vi "Stuck Key Parser.vi"(8 "error in (no error)":errorcluster, 10 "Numeric":u64, 11 "Parser Output Bundle":T1) -> (0 "error out":errorcluster, 3 "output cluster":T1)   [LabVIEW 2016]
panel:
  out "Group 7":bool[](array[boolean])
  out "Group 6":bool[](array[boolean])
  out "Group 5":bool[](array[boolean])
  out "Group 4":bool[](array[boolean])
  out "Group 3":bool[](array[boolean])
  out "Group 2":bool[](array[boolean])
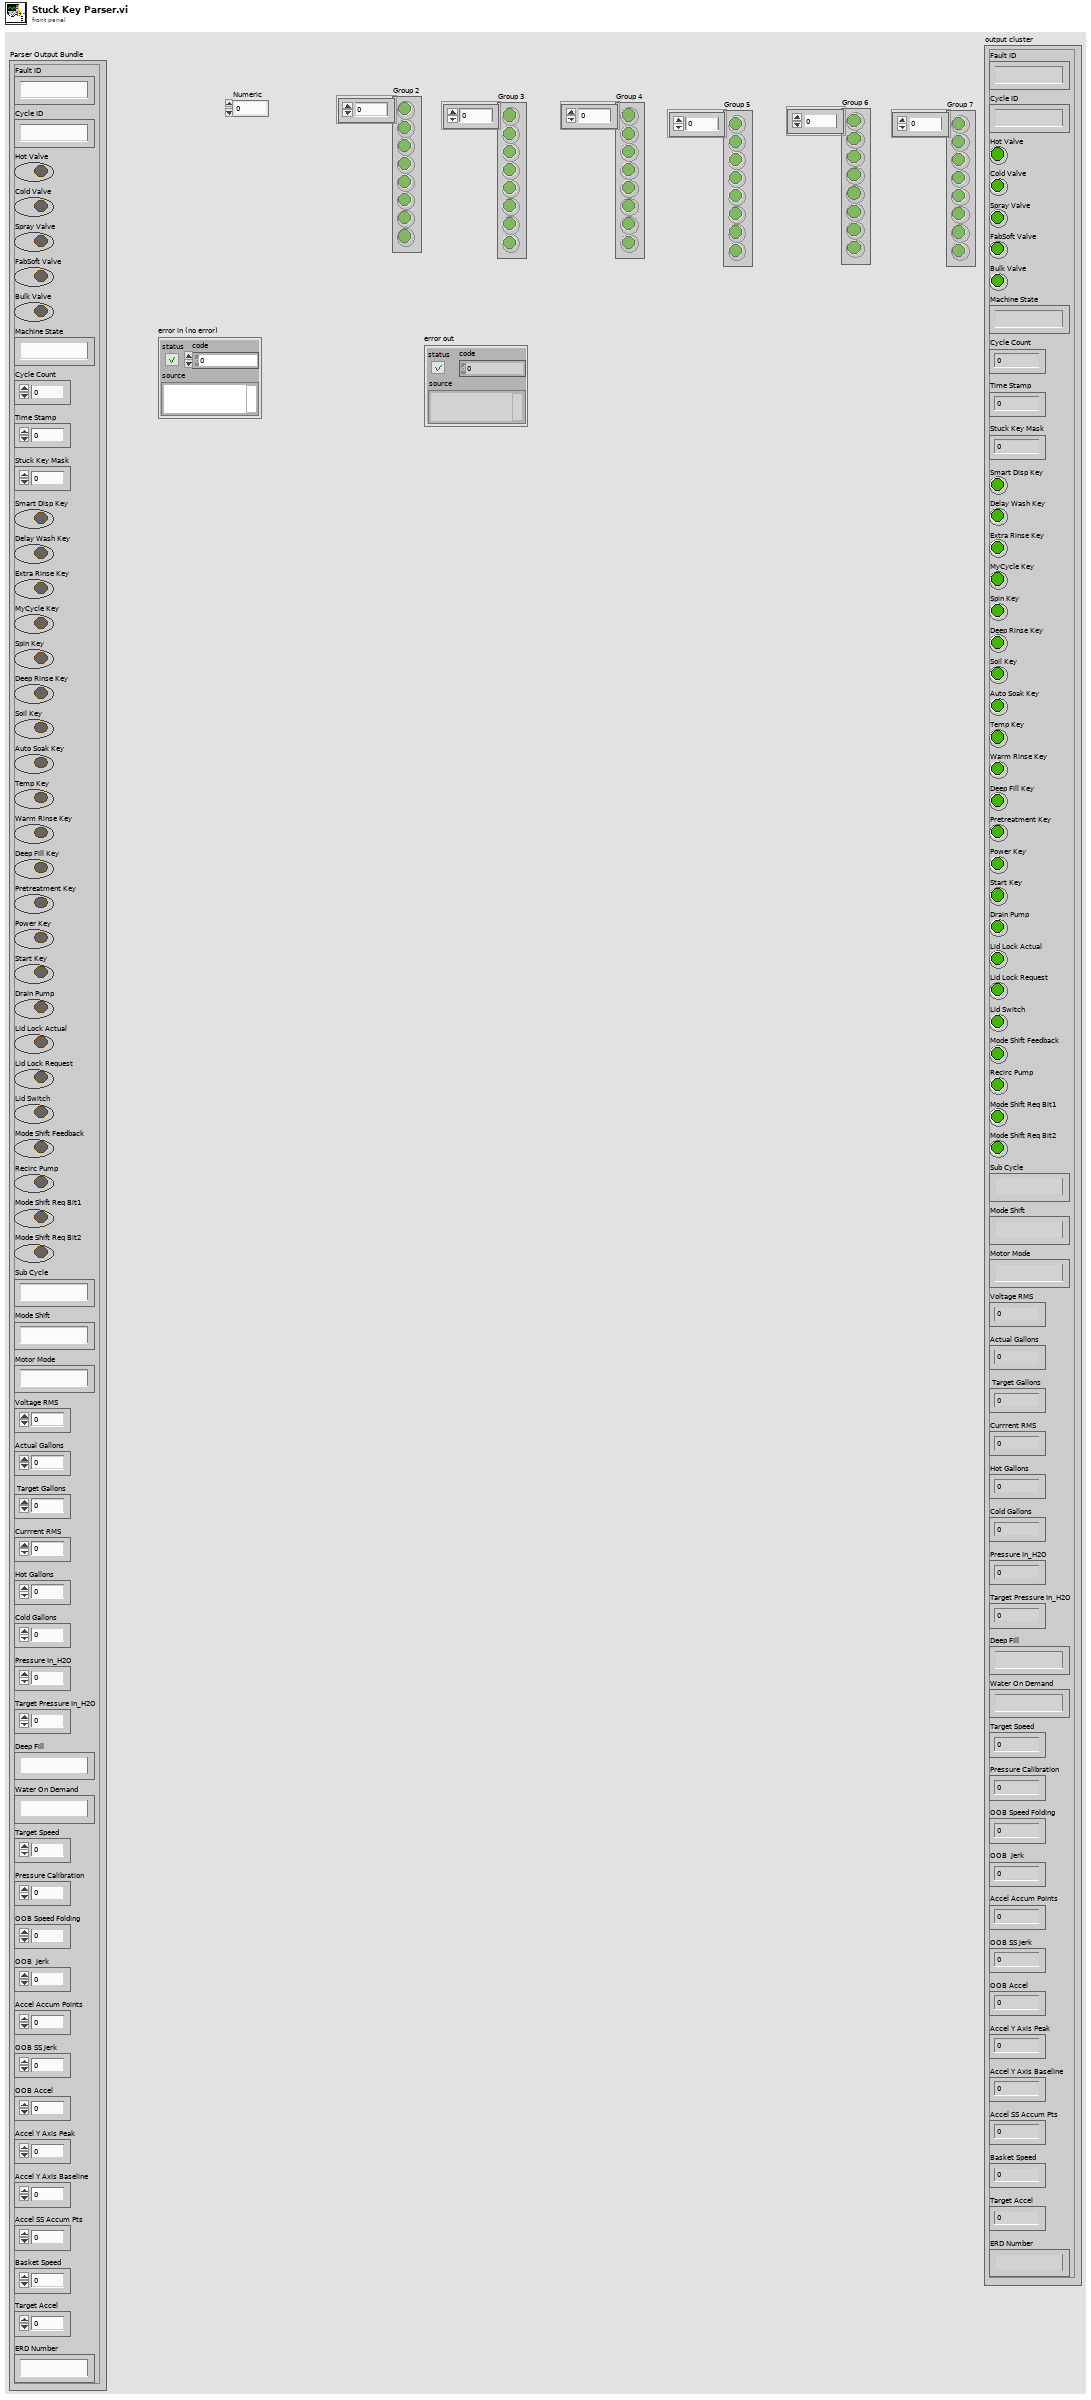
[diagram p1: front panel]
types:
  T1 = cluster{"Fault ID":string, "Cycle ID":string, "Hot Valve":bool, "Cold Valve":bool, "Spray Valve":bool, "FabSoft Valve":bool, "Bulk Valve":bool, "Machine State":string, "Cycle Count":u32, "Time Stamp":u32, "Stuck Key Mask ":u64, "Smart Disp Key":bool, "Delay Wash Key":bool, "Extra Rinse Key":bool, "MyCycle Key":bool, "Spin Key":bool, "Deep Rinse Key":bool, "Soil Key":bool, "Auto Soak Key":bool, "Temp Key":bool, "Warm Rinse Key":bool, "Deep Fill Key":bool, "Pretreatment Key":bool, "Power Key":bool, "Start Key":bool, "Drain Pump":bool, "Lid Lock Actual":bool, "Lid Lock Request":bool, "Lid Switch":bool, "Mode Shift Feedback":bool, "Recirc Pump":bool, "Mode Shift Req Bit1":bool, "Mode Shift Req Bit2":bool, "Sub Cycle":string, "Mode Shift":string, "Motor Mode":string, "Voltage RMS":u16, "Actual Gallons":u16, " Target Gallons":u16, "Currrent RMS":u16, "Hot Gallons":u16, "Cold Gallons":u16, "Pressure In_H2O":u32, "Target Pressure In_H2O":dbl, "Deep Fill":string, "Water On Demand":string, "Target Speed":u16, "Pressure Calibration":u32, "OOB Speed Folding":i32, "OOB  Jerk":i32, "Accel Accum Points":u8, "OOB SS Jerk":i32, "OOB Accel":i32, "Accel Y Axis Peak":i16, "Accel Y Axis Baseline":i16, "Accel SS Accum Pts":u8, "Basket Speed":u16, "Target Accel":u16, "ERD Number":string}
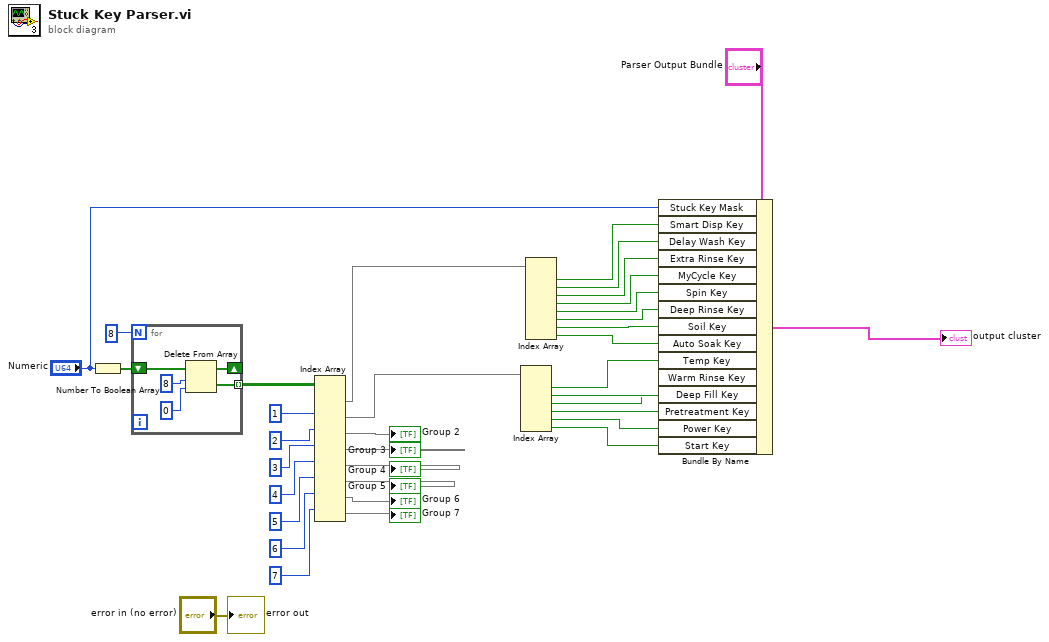
[diagram p0: block diagram]
diagram:
  n1 = Number To Boolean Array(number="Numeric") -> (Boolean array=w29:bool[])
  n2 = for {
    N: 8 -> [_]
    shift-right: [w40] -> _
    shift-left: w29 -> [w41]
    tunnel: [w39] -> w27 mode=indexing
    n3 = Delete From Array(array=w41, length=8, index=0) -> (deleted portion=w39:bool[], array with subset deleted=w40:bool[])
  }
  n4 = Index Array(array=w27, index (row) #2=1 ("index (row)"), index (row) #3=2 ("index (row)"), index (row) #4=3 ("disabled index (col)"), index (row) #5=4 ("disabled index (row)"), index (row) #6=5 ("index (row)"), index (row) #7=6 ("index (row)"), index (row) #8=7 ("index (row)")) -> (element #1=w13:bool[], element #2=w12:bool[], element #3=→"Group 2":bool[], element #4=→"Group 3":bool[], element #5=→"Group 4":bool[], element #6=→"Group 5":bool[], element #7=→"Group 6":bool[], element #8=→"Group 7":bool[])  [unwired: 9 in]
  n5 = Index Array(array=w12) -> (element #1=w7:bool, element #2=w6:bool, element #3=w5:bool, element #4=w4:bool, element #5=w3:bool, element #6=w2:bool)  [unwired: 6 in]
  n6 = Index Array(array=w13) -> (element #1=w34:bool, element #2=w32:bool, element #3=w31:bool, element #4=w30:bool, element #5=w11:bool, element #6=w10:bool, element #7=w9:bool, element #8=w8:bool)  [unwired: 8 in]
  n7 = Bundle By Name(cluster="Parser Output Bundle", "Stuck Key Mask"="Numeric", "Smart Disp Key"=w34, "Delay Wash Key"=w32, "Extra Rinse Key"=w31, "MyCycle Key"=w30, "Spin Key"=w11, "Deep Rinse Key"=w10, "Soil Key"=w9, "Auto Soak Key"=w8, "Temp Key"=w7, "Warm Rinse Key"=w6, "Deep Fill Key"=w5, "Pretreatment Key"=w4, "Power Key"=w3, "Start Key"=w2) -> (→"output cluster":T1)
  "error out" <- "error in (no error)"
